vi "PH_PILS.set Doors Laserbay.vi"(0 "i ref in":refnum<vi>, 2 "Service Name":string="N/A", 5 "error in":errorcluster) -> (14 "i ref out":refnum<vi>, 19 "error out":errorcluster)   [LabVIEW 2014, in "PH_PILS.lvlib"]
doc: "This VI sets the GUI elements related to the doors at the laserbay."
uses:
  PH_PILS.lvlib
  PH_PILS.Operation Mode.ctl
  PH_Common/PH_Common.lvlib
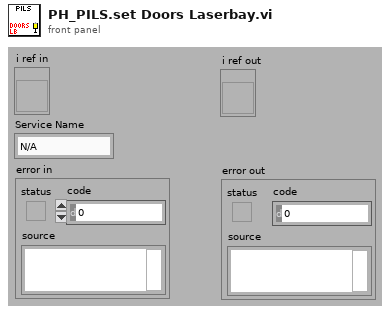
[diagram p1: front panel]
types:
  T1 = typedef "PH_PILS.lvlib/PH_PILS.Operation Mode.ctl" = enum16{"unknown", "Service", "Labor", "Search", "Shot"}
  T2 = typedef "PH_PILS.lvlib/PH_PILS.i attribute.ctl" = cluster{"Boolean":cluster{"GUI Ref":refnum<vi>, "Status":i32}[], "GUI Refs Exp. Shutters":cluster{"1":refnum<vi>, "2":refnum<vi>, "3":refnum<vi>, "4":refnum<vi>}, "Tristate2Run GUI Refs":refnum<vi>[], "EO-Likes":cluster{"GUI Ref":refnum<vi>, "Status":i32}[], "Operation Mode":cluster{"Operation Mode":T1, "GUI":cluster{"Ref State":refnum<vi>, "Ref":refnum<vi>}, "Servicemode":cluster{"Tagname":string, "Status":i32}, "Labormode":cluster{"Tagname":string, "Status":i32}, "Searchmode":cluster{"Tagname":string, "Status":i32}, "Shotmode":cluster{"Tagname":string, "Status":i32}}, "Submode":cluster{"Submode":T3, "GUI":cluster{"Ref State":refnum<vi>, "Ref":refnum<vi>}, "Submode":cluster{"Tagname":string, "Status":i32}}, "Experiment":cluster{"Experiment":enum16{"unknown", "intern", "4 (Z6)", "3", "2", "1"}, "GUI":cluster{"Ref State":refnum<vi>, "Ref":refnum<vi>}, "intern":cluster{"Tagname":string, "Status":i32}, "Exp 4":cluster{"Tagname":string, "Status":i32}, "Exp 3":cluster{"Tagname":string, "Status":i32}, "Exp 2":cluster{"Tagname":string, "Status":i32}, "Exp 1":cluster{"Tagname":string, "Status":i32}}, "TristateNormal":cluster{"GUI Ref":refnum<vi>, "Status":i32}[], "Door Tags":cluster{"GUI Ref":refnum<vi>, "Status":i32}[], "GUIlessTags":cluster{"Name":string, "Status":i32}[], "Beamline GUI Refs":refnum<vi>[], "Special Boolean":cluster{"GUI Ref":refnum<vi>, "Status":i32}[], "Laserpower":cluster{"GUI Ref":refnum<vi>, "Status":i32}[], "Shutter":cluster{"GUI Ref":refnum<vi>, "Status":i32}[], "Tristate EO Like":cluster{"GUI Ref":refnum<vi>, "Status":i32}[], "PP":cluster{"GUI Ref":refnum<vi>, "Status":i32, "Head Ref":refnum<vi>, "Slider Ref":refnum<vi>}[], "Switch Knobs":cluster{"GUI Ref":refnum<vi>, "Status":i32}[], "Latch Knob GUI Refs":refnum<vi>[], "FailureCounter":i32, "Enabled Status":cluster{"Laser":i32, "PreAmp":i32, "MainAmp":i32}, "Mercury":refnum<vi>, "Instance Rods":string, "Logfile":path, "Beckhoff-Instance Internal":string, "Beckhoff-Instance External":string, "Enabling Rights":cluster{"Name":string, "Password":string, "PA?":bool, "MA?":bool, "Exp?":bool}[]}
  T3 = typedef "PH_PILS.lvlib/PH_PILS.Submode.ctl" = enum16{"unknown", "HV-Normal", "HV-Test"}
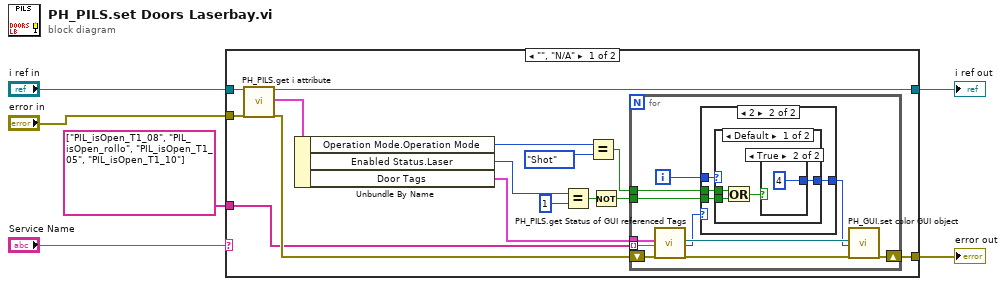
[diagram p0: block diagram]
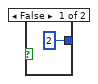
[diagram p3: hidden frame]
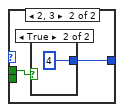
[diagram p4: hidden frame]
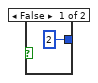
[diagram p5: hidden frame]
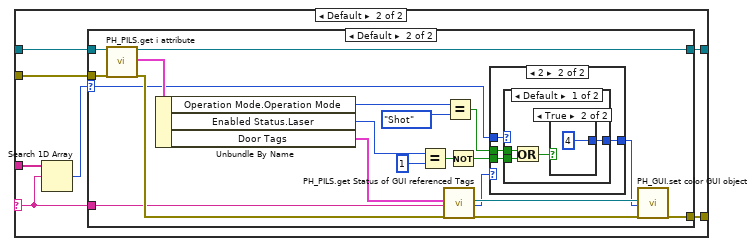
[diagram p6: hidden frame]
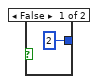
[diagram p9: hidden frame]
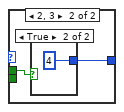
[diagram p10: hidden frame]
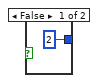
[diagram p11: hidden frame]
diagram:
  n1 = case shown="\"\", \"N/A\"" "Service Name" {
    selector: "Service Name" -> [_ w50]
    tunnel: "error in" -> [w21 w54]
    tunnel: [w20 w53] -> w5
    tunnel: "i ref in" -> [w19 w52]
    tunnel: [w17 w51] -> w3
    tunnel: string[] ["PIL_isOpen_T1_08", "PIL_isOpen_rollo", "PIL_isOpen_T1_05", "PIL_isOpen_T1_10"] -> [w7 w48]
    frame "", "N/A" {
      n2 = call "PH_PILS.get i attribute.vi"("i ref in"=w19, "error in (no error)"=w21) -> ("i ref out"=w20:refnum<vi>, "i attribute"=w18:T2, "error out"=w8:errorcluster)  [unwired: 15 in]
      n3 = Unbundle By Name(w18) -> ("Operation Mode.Operation Mode"=w16:T1, "Enabled Status.Laser"=w14:i32, "Door Tags"=w9:cluster{"GUI Ref":refnum<vi>, "Status":i32}[])
      n4 = Equal?(x=w14, y=1) -> (x = y?=w12:bool)
      n5 = Equal?(x=w16, y=PH_PILS.Operation_Mode."Shot" ("Operation Mode.Operation Mode")) -> (x = y?=w10:bool)
      n6 = Not(x=w12) -> (.not. x?=w11:bool)
      n7 = for {
        tunnel: w9 -> [w32]
        tunnel: w7 -> [w29] mode=indexing
        shift-right: [w28] -> w17
        shift-left: w8 -> [w31]
        tunnel: w11 -> [w23]
        tunnel: w10 -> [w22]
        i -> [w24]
        n8 = call "PH_PILS.get Status of GUI referenced Tags.vi"("Tags"=w32, "Tagname"=w29, "error in"=w31) -> ("GUI Ref"=w27:refnum<vi>, "Status"=w26:i32, "error out"=w30:errorcluster)  [unwired: 13 in, 1 out]
        n9 = case shown="2" w26 {
          selector: w26 -> [w33 _]
          tunnel: [w33 w36] -> w25
          tunnel: w24 -> [_ w37]
          tunnel: w23 -> [_ w35]
          tunnel: w22 -> [_ w34]
          frame 0, Default {
          }
          frame 2 {
            n10 = case shown="Default" w37 {
              tunnel: [w41 w45] -> w36
              tunnel: w35 -> [w40 _]
              tunnel: w34 -> [w38 w44]
              frame Default {
                n11 = Or(x=w38, y=w40) -> (x .or. y?=w39:bool)
                n12 = case shown="True" w39 {
                  tunnel: [2 4] -> w41
                  frame False {
                  }
                  frame True {
                  }
                }
              }
              frame 2, 3 {
                n13 = case shown="True" w44 {
                  tunnel: [2 4] -> w45
                  frame False {
                  }
                  frame True {
                  }
                }
              }
            }
          }
        }
        n14 = call "PH_GUI.set color GUI object.vi"("GUI object Ref"=w27, "State"=w25, "error in (no error)"=w30) -> ("error out"=w28:errorcluster)  [unwired: 16 in]
      }
    }
    frame Default {
      n15 = Search 1D Array(1D array=w48, element=w50) -> (index of element=w49:i32)  [unwired: 1 in]
      n16 = case shown="Default" w49 {
        selector: w49 -> [_ w57]
        tunnel: w54 -> [w55 w76]
        tunnel: [w56 w75] -> w53
        tunnel: w52 -> [w56 w74]
        tunnel: [w55 w72] -> w51
        tunnel: w50 -> [_ w62]
        frame -1 {
        }
        frame Default {
          n17 = call "PH_PILS.get i attribute.vi"("i ref in"=w74, "error in (no error)"=w76) -> ("i ref out"=w75:refnum<vi>, "i attribute"=w73:T2, "error out"=w63:errorcluster)  [unwired: 15 in]
          n18 = Unbundle By Name(w73) -> ("Operation Mode.Operation Mode"=w71:T1, "Enabled Status.Laser"=w69:i32, "Door Tags"=w64:cluster{"GUI Ref":refnum<vi>, "Status":i32}[])
          n19 = Equal?(x=w69, y=1) -> (x = y?=w67:bool)
          n20 = call "PH_PILS.get Status of GUI referenced Tags.vi"("Tags"=w64, "Tagname"=w62, "error in"=w63) -> ("GUI Ref"=w60:refnum<vi>, "Status"=w59:i32, "error out"=w61:errorcluster)  [unwired: 13 in, 1 out]
          n21 = Equal?(x=w71, y=PH_PILS.Operation_Mode."Shot" ("Operation Mode.Operation Mode")) -> (x = y?=w65:bool)
          n22 = Not(x=w67) -> (.not. x?=w66:bool)
          n23 = case shown="2" w59 {
            selector: w59 -> [w77 _]
            tunnel: [w77 w80] -> w58
            tunnel: w57 -> [_ w81]
            tunnel: w66 -> [_ w79]
            tunnel: w65 -> [_ w78]
            frame 0, Default {
            }
            frame 2 {
              n24 = case shown="Default" w81 {
                tunnel: [w85 w89] -> w80
                tunnel: w79 -> [w84 _]
                tunnel: w78 -> [w82 w88]
                frame Default {
                  n25 = Or(x=w82, y=w84) -> (x .or. y?=w83:bool)
                  n26 = case shown="True" w83 {
                    tunnel: [2 4] -> w85
                    frame False {
                    }
                    frame True {
                    }
                  }
                }
                frame 2, 3 {
                  n27 = case shown="True" w88 {
                    tunnel: [2 4] -> w89
                    frame False {
                    }
                    frame True {
                    }
                  }
                }
              }
            }
          }
          n28 = call "PH_GUI.set color GUI object.vi"("GUI object Ref"=w60, "State"=w58, "error in (no error)"=w61) -> ("error out"=w72:errorcluster)  [unwired: 16 in]
        }
      }
    }
  }
  "error out" <- w3
  "i ref out" <- w5
